vi "OAT Multistage Decimation with IC.vi"(6 "initial state":cluster{"initial state":dbl[]}[](array[cluster]) {"initial state" format="%.2f"}, 8 "error in (no error)":errorcluster, 9 "filter":T1[](array[typedef]) {"coefficients" format="%.2f"}, 11 "X":dbl[](array[numeric]) format="%.2f") -> (0 "error out":errorcluster, 3 "Y":dbl[](array[numeric]) format="%.2f", 4 "final state":cluster{"final state":dbl[]}[](array[cluster]) {"final state" format="%.2f"})   [LabVIEW 2017, in "SoundVib_Resampling.lvlib"]
doc: "Decimate the input sequence <B>X</B> with the multistage decimation filter specified by <B>filter</B>."
uses:
  <vilib>/addons/Sound and Vibration/Order Analysis/Resample Order Tracking/SoundVib_Resampling.lvlib
  <vilib>/addons/_NISVFA/_Shared subVIs/Controls/OAT Decimation Filter.ctl
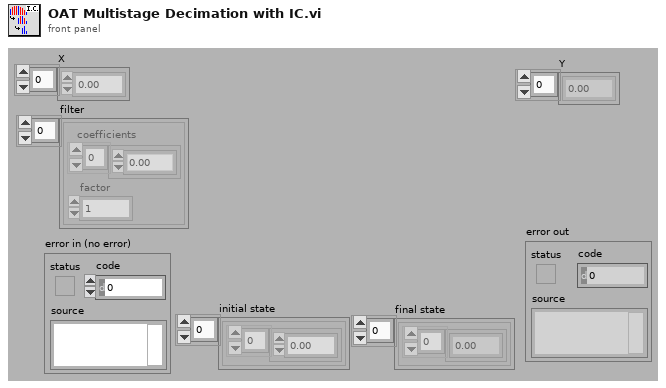
[diagram p1: front panel]
types:
  T1 = typedef "OAT Decimation Filter.ctl" = cluster{"coefficients":dbl[], "factor":i32}
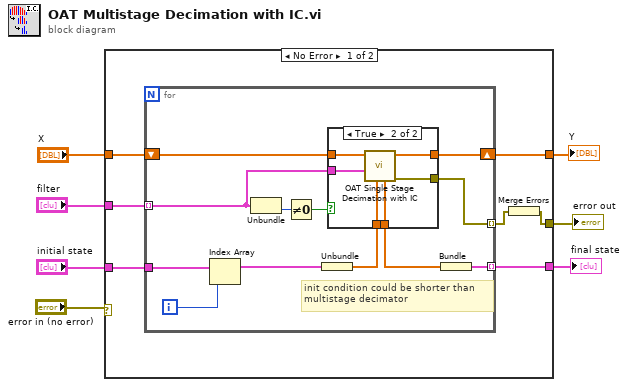
[diagram p0: block diagram]
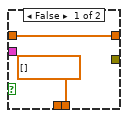
[diagram p2: hidden frame]
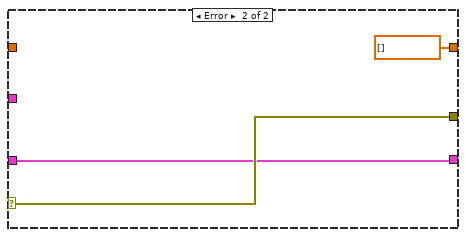
[diagram p3: hidden frame]
diagram:
  n1 = case shown="No Error" "error in (no error)" {
    selector: "error in (no error)" -> [_ w37]
    tunnel: "X" -> [w14 _]
    tunnel: [w13 w36] -> w6
    tunnel: [w12 dbl[] [] ("X")] -> w5
    tunnel: "initial state" -> [w11 w36]
    tunnel: "filter" -> [w10 _]
    tunnel: [w8 w37] -> w2
    frame No Error {
      n2 = for {
        shift-right: [w23] -> w12
        shift-left: w14 -> [w24]
        tunnel: [w21] -> w13 mode=indexing
        tunnel: w11 -> [w19]
        tunnel: w10 -> [w16] mode=indexing
        tunnel: [w15] -> w9 mode=indexing
        i -> [w18]
        # "init condition could be shorter than \nmultistage decimator"
        n3 = Index Array(array=w19, index=w18) -> (element=w17:cluster{"initial state":dbl[]})
        n4 = Unbundle(w16) -> ("factor"=w26:i32)  [unwired: 1 out]
        n5 = Not Equal To 0?(x=w26) -> (x != 0?=w25:bool)
        n6 = Unbundle(w17) -> ("initial state"=w20:dbl[])
        n7 = case shown="True" w25 {
          tunnel: w24 -> [w28 w34]
          tunnel: w16 -> [_ w33]
          tunnel: [w28 w32] -> w23
          tunnel: [dbl[] [] ("final condition") w31] -> w22
          tunnel: w20 -> [_ w30]
          tunnel: [_ w29] -> w15
          frame False {
          }
          frame True {
            n8 = call <vilib>:"OAT Single Stage Decimation with IC.vi"("initial state"=w30, "filter"=w33, "X"=w34) -> ("error out"=w29:errorcluster, "Y"=w32:dbl[], "final state"=w31:dbl[])  [unwired: 6 in]
          }
        }
        n9 = Bundle("final state"=w22) -> (w21:cluster{"final state":dbl[]})  [unwired: 1 in]
      }
      n10 = Merge Errors(w9) -> (w8:errorcluster)
    }
    frame Error {
    }
  }
  "Y" <- w5
  "final state" <- w6
  "error out" <- w2
